vi "Script_Timing_Extract_Total_Duration.vi"(8 "error in (no error)":errorcluster, 11 "Script":string="\r\n") -> (0 "error out":errorcluster, 3 "Total duration (s)":i32)   [LabVIEW 2018]
panel:
  out "Repeats":i32
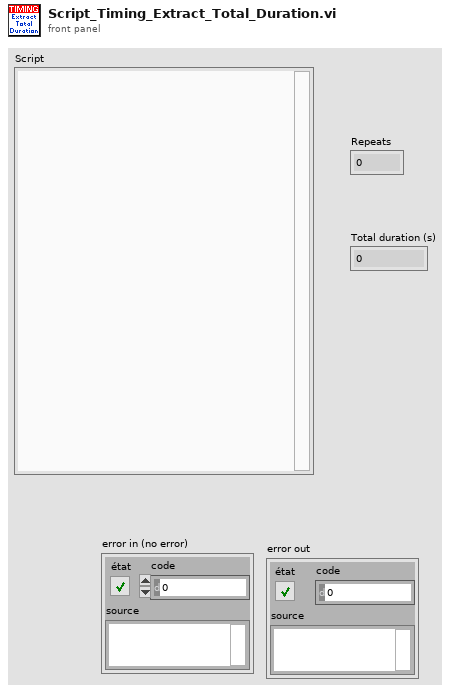
[diagram p1: front panel]
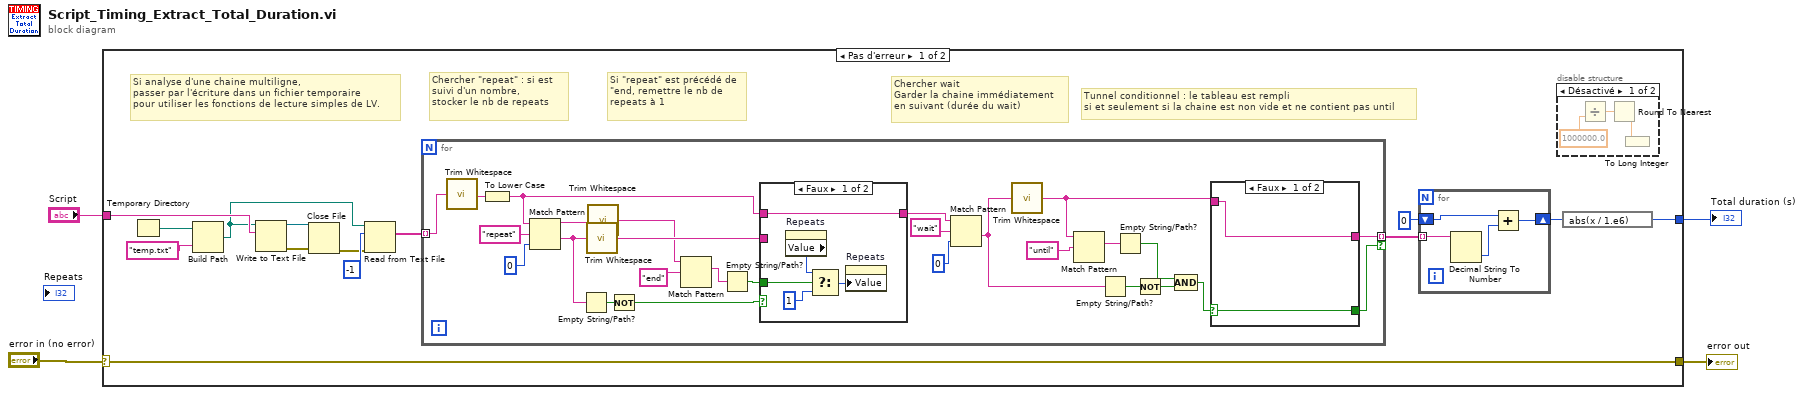
[diagram p0: block diagram]
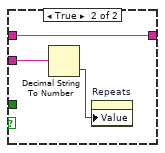
[diagram p3: hidden frame]
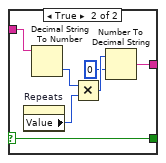
[diagram p4: hidden frame]
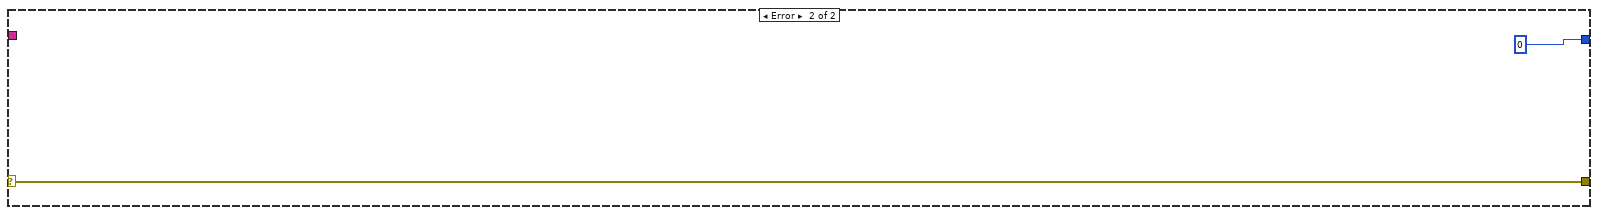
[diagram p5: hidden frame]
diagram:
  n1 = case shown="Pas d'erreur" "error in (no error)" {
    selector: "error in (no error)" -> [w18 w71]
    tunnel: [w18 w71] -> w3
    tunnel: "Script" -> [w15 _]
    tunnel: [w5 0] -> w1
    frame No Error {
      # "Si \"repeat\" est précédé de \"end, remettre le nb de repeats à 1"
      # "Chercher \"repeat\" : si est suivi d'un nombre,\nstocker le nb de repeats"
      # "Si analyse d'une chaine multiligne,\npasser par l'écriture dans un fichier temporaire\npour utiliser les fonctions de lecture simples de LV."
      # "Tunnel conditionnel : le tableau est rempli\nsi et seulement si la chaine est non vide et ne contient pas until"
      # "Chercher wait\nGarder la chaine immédiatement\nen suivant (durée du wait)"
      n2 = Temporary Directory() -> (w16:path)
      n3 = Build Path(base path=w16, name or relative path="temp.txt" ("nom ou chemin relatif")) -> (appended path=w12:path)
      n4 = Write to Text File(file (use dialog)=w12, text=w15) -> (refnum out=w13:refnum<file>, error out=w14:errorcluster)  [unwired: 2 in, 1 out]
      n5 = Close File(refnum=w13, error in=w14) -> (error out=w9:errorcluster)  [unwired: 1 out]
      n6 = Read from Text File(file (use dialog)=w12, count=-1 ("nombre"), error in=w9) -> (text=w10:string[])  [unwired: 1 in, 3 out]
      n7 = for {
        tunnel: w10 -> [w52] mode=indexing
        tunnel: [w27] -> w7 mode=indexing if=w26
        n8 = call <vilib>:"Trim Whitespace.vi"("string"=w52) -> ("trimmed string"=w43:string)  [unwired: 1 in]
        n9 = To Lower Case(string=w43) -> (all lower case string=w35:string)
        n10 = Match Pattern(string=w35, regular expression="repeat" ("expression régulière"), offset (0)=0) -> (before substring=w32:string, after substring=w38:string)  [unwired: 2 out]
        n11 = Empty String/Path?(string/path=w38) -> (empty?=w39:bool)
        n12 = call <vilib>:"Trim Whitespace.vi"("string"=w38) -> ("trimmed string"=w40:string)  [unwired: 1 in]
        n13 = call <vilib>:"Trim Whitespace.vi"("string"=w32) -> ("trimmed string"=w30:string)  [unwired: 1 in]
        n14 = Not(x=w39) -> (.not. x?=w37:bool)
        n15 = Match Pattern(string=w30, regular expression="end" ("expression régulière")) -> (match substring=w28:string)  [unwired: 1 in, 3 out]
        n16 = Empty String/Path?(string/path=w28) -> (empty?=w31:bool)
        n17 = case shown="Faux" w37 {
          tunnel: w40 -> [_ w60]
          tunnel: [w57 w59] -> w36
          tunnel: w35 -> [w57 w59]
          tunnel: w31 -> [w56 _]
          frame False {
            n18 = property on="Repeats" class="NumNb (strict)"() -> ("Value"=w53:i32)  [unwired: 2 in, 2 out]
            n19 = Select(t=w53, s=w56, f=1 ("nombre")) -> (s? t:f=w54:i32)
            n20 = property on="Repeats" class="NumNb (strict)"("Value"=w54) -> ()  [unwired: 2 in, 2 out]
          }
          frame True {
            n21 = Decimal String To Number(string=w60) -> (number=w58:i32)  [unwired: 2 in, 1 out]
            n22 = property on="Repeats" class="NumNb (strict)"("Value"=w58) -> ()  [unwired: 2 in, 2 out]
          }
        }
        n23 = Match Pattern(string=w36, regular expression="wait" ("expression régulière"), offset (0)=0) -> (after substring=w48:string)  [unwired: 3 out]
        n24 = call <vilib>:"Trim Whitespace.vi"("string"=w48) -> ("trimmed string"=w33:string)  [unwired: 1 in]
        n25 = Match Pattern(string=w33, regular expression="until" ("expression régulière")) -> (match substring=w45:string)  [unwired: 1 in, 3 out]
        n26 = Empty String/Path? ("Chemin/Chaîne vide ?")(string/path=w48) -> (empty?=w49:bool)
        n27 = Empty String/Path? ("Chemin/Chaîne vide ?")(string/path=w45) -> (empty?=w44:bool)
        n28 = Not(x=w49) -> (.not. x?=w46:bool)
        n29 = Compound Arithmetic op=AND ("Opérateur arithmétique")(w44, w46) -> (w34:bool)
        n30 = case shown="Faux" w34 {
          selector: w34 -> [w61 w64]
          tunnel: w33 -> [w62 w69]
          tunnel: [w62 w65] -> w27
          tunnel: [w61 w64] -> w26
          frame False {
          }
          frame True {
            n31 = property on="Repeats" class="NumNb (strict)"() -> ("Value"=w67:i32)  [unwired: 2 in, 2 out]
            n32 = Decimal String To Number(string=w69) -> (number=w68:i32)  [unwired: 2 in, 1 out]
            n33 = Multiply(x=w68, y=w67) -> (x*y=w66:i32)
            n34 = Number To Decimal String(number=w66, width (-)=0 ("largeur (-)")) -> (decimal integer string=w65:string)
          }
        }
      }
      n35 = for {
        tunnel: w7 -> [w22] mode=indexing
        shift-right: [w25] -> w6
        shift-left: 0 -> [w23]
        n36 = Decimal String To Number(string=w22) -> (number=w24:i32)  [unwired: 2 in, 1 out]
        n37 = Add(x=w23, y=w24) -> (x+y=w25:i32)
      }
      n38 = disable-structure shown="Désactivé" {
        frame Disabled {
          n39 = Divide(y=1000000.0) -> (x/y=w20:dbl)  [unwired: 1 in]
          n40 = Round To Nearest(number=w20) -> (nearest integer value=w19:dbl)
          n41 = To Long Integer(number=w19) -> ()  [unwired: 1 out]
        }
        frame Enabled {
        }
      }
      n42 = expression code="abs(x / 1.e6)"(w6) -> (w5:i32)
    }
    frame Error {
    }
  }
  "error out" <- w3
  "Total duration (s)" <- w1
